vi "ElevatorBegin.vi"(8 "error in (no error)":errorcluster) -> (0 "error out":errorcluster)   [LabVIEW 2023]
doc: "Opens and sets up two SPARK Max Motor Controllers and two limit switches for the Elevator\n\nInputs:\n--Error in--cluster\n\nOutputs:\n--Error out--cluster"
uses:
  <vilib>/Rock Robotics/SystemInterfaces/DIO/FPGA_DIOChannel.ctl
  <vilib>/Rock Robotics/WPI/ThirdParty/REV Robotics/REVLib/Typedef/Spark MAX Limit Switch Polarity.ctl
  <vilib>/Rock Robotics/WPI/ThirdParty/REV Robotics/REVLib/Typedef/Spark MAX Limit Direction.ctl
  <vilib>/Rock Robotics/WPI/ThirdParty/REV Robotics/REVLib/Typedef/Spark MAX Idle Mode.ctl
  <vilib>/Rock Robotics/WPI/ThirdParty/REV Robotics/REVLib/Typedef/Spark MAX Motor Type.ctl
  <vilib>/Rock Robotics/WPI/ThirdParty/REV Robotics/REVLib/Typedef/Spark MAX Sensor Type.ctl
  <vilib>/Rock Robotics/WPI/Switch/WPI_SwitchOpenLimit.vi
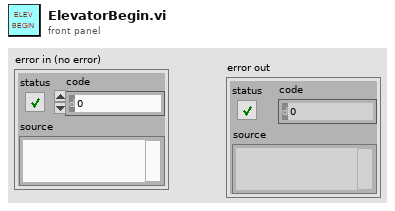
[diagram p1: front panel]
types:
  T1 = typedef "FPGA_DIOChannel.ctl" = enum8{"DIO 0", "DIO 1", "DIO 2", "DIO 3", "DIO 4", "DIO 5", "DIO 6", "DIO 7", "DIO 8", "DIO 9", "DIO MXP 0", "DIO MXP 1", "DIO MXP 2", "DIO MXP 3", "DIO MXP 4", "DIO MXP 5", "DIO MXP 6", "DIO MXP 7", "DIO MXP 8", "DIO MXP 9", "DIO MXP 10", "DIO MXP 11", "DIO MXP 12", "DIO MXP 13", "DIO MXP 14", "DIO MXP 15", "SPI Port CS1", "SPI Port CS2", "SPI Port CS3", "SPI Port MISO", "SPI Port MOSI", "Invalid"}
  T2 = typedef "Spark MAX Limit Switch Polarity.ctl" = enum16{"Normally Open", "Normally Closed"}
  T3 = typedef "Spark MAX Limit Direction.ctl" = enum16{"Forward Limit", "Reverse Limit"}
  T4 = typedef "Spark MAX Idle Mode.ctl" = enum16{"Coast", "Brake"}
  T5 = typedef "Spark MAX Motor Type.ctl" = enum16{"Brushed", "Brushless"}
  T6 = typedef "Spark MAX Sensor Type.ctl" = enum16{"No Sensor", "Hall Sensor", "Encoder", "-Not Available-", "Analog", "Alternate Encoder", "Duty Cycle"}
  T7 = typedef "WPI_MotorControlDeviceRef.ctl" = cluster{"DeviceStatus":errorcluster, "Type":T8, "PWM":cluster{"PWM Channel":T9, "DeadBand":T10}, "CAN":cluster{"Device Number":u8, "SetOutput VI Ref":variant, "GetOutput VI Ref":variant, "Enable VI Ref":variant, "Disable VI Ref":variant, "Data":variant}, "Invert":bool, "DIO PWM":cluster{"PWM \"Enable\" Channel":T9, "DIOChannel":T1, "PWM Rate":dbl}}
  T8 = typedef "WPI_MotorControlType.ctl" = enum16{"PWM", "CAN", "DIO PWM"}
  T9 = typedef "FPGA_DIOPWMChannel.ctl" = enum8{"PWM 0", "PWM 1", "PWM 2", "PWM 3", "PWM 4", "PWM 5", "PWM 6", "PWM 7", "PWM 8", "PWM 9", "PWM MXP 0", "PWM MXP 1", "PWM MXP 2", "PWM MXP 3", "PWM MXP 4", "PWM MXP 5", "PWM MXP 6", "PWM MXP 7", "PWM MXP 8", "PWM MXP 9", "Invalid"}
  T10 = typedef "WPI_PWMDeadband.ctl" = cluster{"Name":string, "maxPositivePwm":i32, "minPositivePwm":i32, "centerPwm":i32, "maxNegativePwm":i32, "minNegativePwm":i32, "angularRange":u16}
  T11 = typedef "WPI_SwitchDevRef.ctl" = cluster{"DevStatus":errorcluster, "DIO Channel":T1, "CntIndex":T12, "Normally Closed":bool}
  T12 = typedef "FPGA_CounterCtrSystemIndex.ctl" = enum8{"Ctr 0", "Ctr 1", "Ctr 2", "Ctr 3", "Ctr 4", "Ctr 5", "Ctr 6", "Ctr 7", "Invalid"}
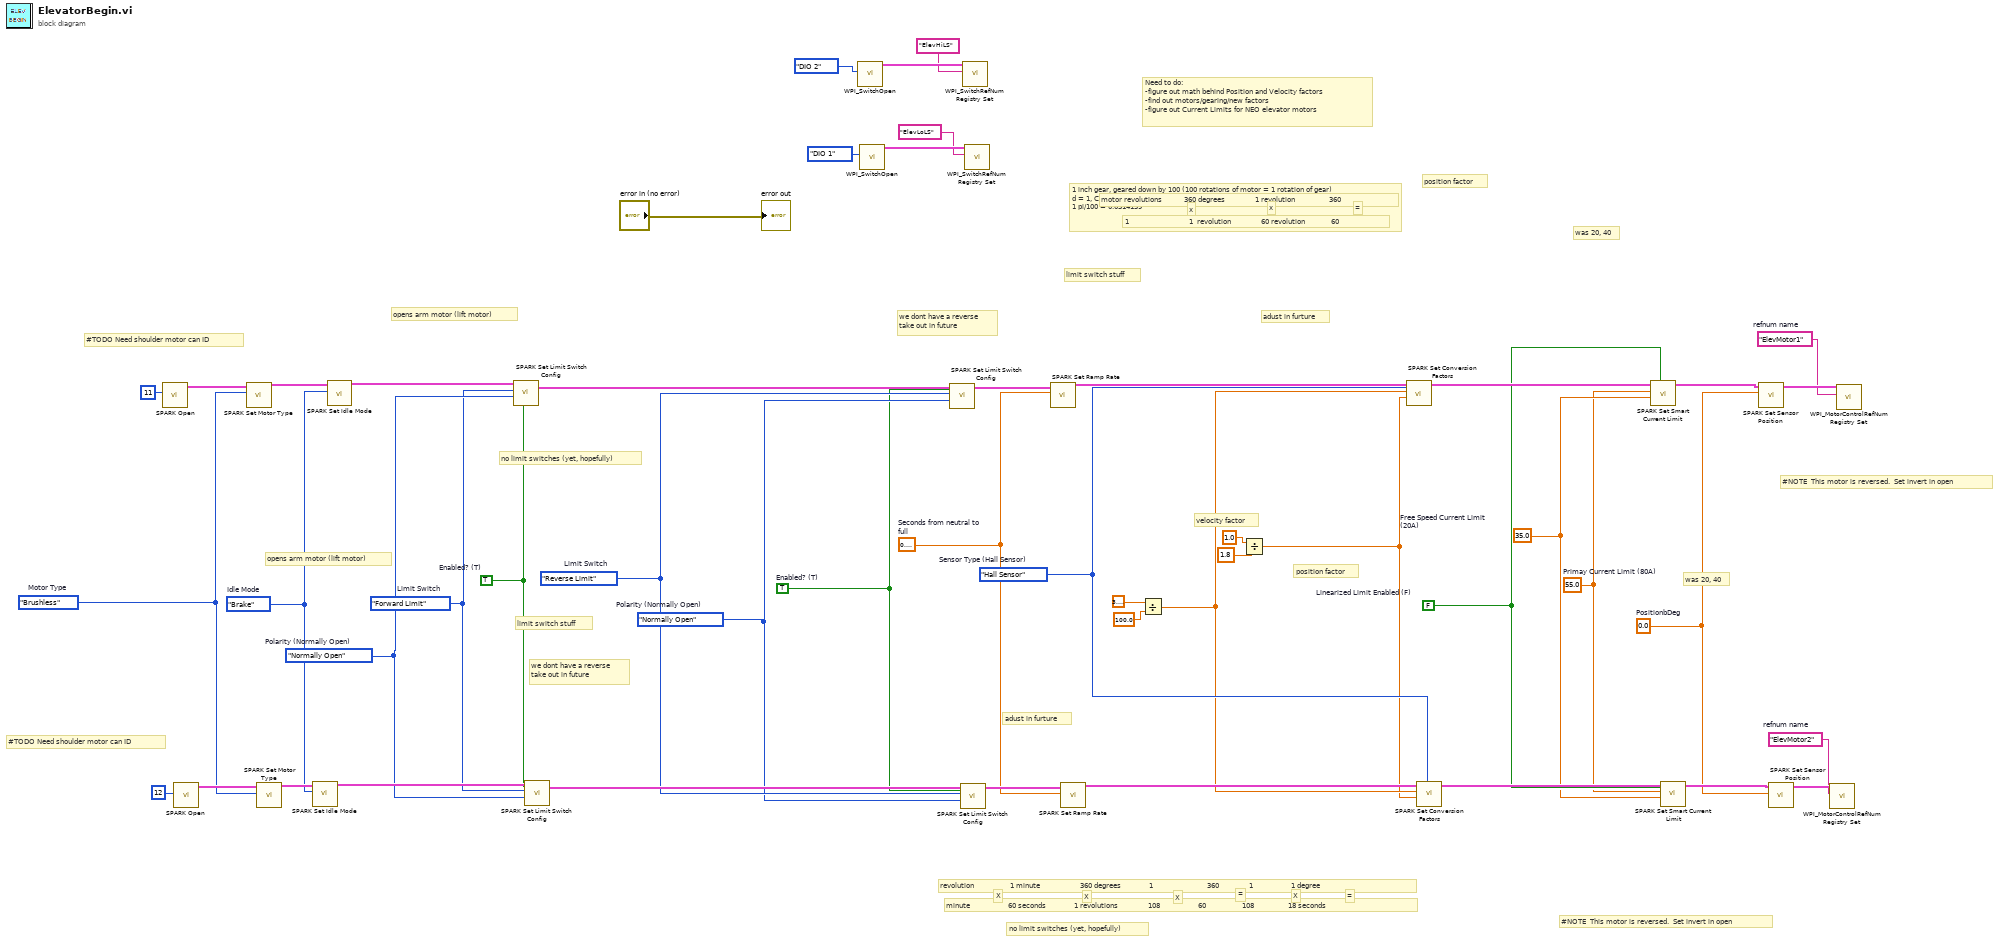
[diagram p0: block diagram]
diagram:
  w4 = FALSE  # Linearized Limit Enabled (F)
  w10 = Spark_MAX_Limit_Switch_Polarity."Normally Open"  # Polarity (Normally Open)
  w11 = Spark_MAX_Limit_Direction."Reverse Limit"  # Limit Switch
  w14 = Spark_MAX_Limit_Switch_Polarity."Normally Open"  # Polarity (Normally Open)
  w13 = Spark_MAX_Limit_Direction."Forward Limit"  # Limit Switch
  w1 = 0.0  # PositionbDeg
  w28 = "ElevMotor2"  # refnum name
  w2 = 55.0  # Primay Current Limit (80A)
  w15 = Spark_MAX_Idle_Mode."Brake"  # Idle Mode
  w16 = Spark_MAX_Motor_Type."Brushless"  # Motor Type
  w7 = Spark_MAX_Sensor_Type."Hall Sensor"  # Sensor Type (Hall Sensor)
  w8 = sgl 0.2  # Seconds from neutral to full
  w9 = TRUE  # Enabled? (T)
  w12 = TRUE  # Enabled? (T)
  w40 = "ElevMotor1"  # refnum name
  w3 = 35.0  # Free Speed Current Limit (20A)
  # "1 inch gear, geared down by 100 (100 rotations of motor = 1 rotation of gear)\nd = 1, C = pi*d = 1pi\n1 pi/100 = 0.0314159"
  # "Need to do: \n-figure out math behind Position and Velocity factors\n-find out motors/gearing/new factors\n-figure out Current Limits for NEO elevator motors"
  # "#NOTE  This motor is reversed.  Set invert in open"
  # "#TODO Need shoulder motor can ID"
  # "no limit switches (yet, hopefully)"
  # "was 20, 40"
  # "we dont have a reverse\ntake out in future"
  # "adust in furture"
  # "position factor"
  # "limit switch stuff"
  # "X"
  # "X"
  # "X"
  # "X"
  # "="
  # "="
  # "minute                   60 seconds              1 revolutions               108                   60                  108                 18 seconds"
  # "revolution                  1 minute                    360 degrees              1                           360               1                   1 degree"
  # "opens arm motor (lift motor)"
  # "#NOTE  This motor is reversed.  Set invert in open"
  # "#TODO Need shoulder motor can ID"
  # "no limit switches (yet, hopefully)"
  # "was 20, 40"
  # "we dont have a reverse\ntake out in future"
  # "adust in furture"
  # "velocity factor"
  # "position factor"
  # "limit switch stuff"
  # "1                              1  revolution               60 revolution             60"
  # "="
  # "x"
  # "x"
  # "motor revolutions           360 degrees               1 revolution                 360"
  # "opens arm motor (lift motor)"
  n1 = call <vilib>:"SPARK Open.vi"("Device Number"=u8 11) -> ("MotorControlDeviceRef"=w44:T7)  [unwired: 9 in, 1 out]
  n2 = call <vilib>:"SPARK Open.vi"("Device Number"=u8 12) -> ("MotorControlDeviceRef"=w32:T7)  [unwired: 9 in, 1 out]
  n3 = call <vilib>:"SPARK Set Motor Type.vi"("Motor Type"=w16, "MotorControlDevRef"=w44) -> ("MotorControlDeviceRef"=w43:T7)  [unwired: 8 in, 1 out]
  n4 = call <vilib>:"SPARK Set Motor Type.vi"("Motor Type"=w16, "MotorControlDevRef"=w32) -> ("MotorControlDeviceRef"=w31:T7)  [unwired: 8 in, 1 out]
  n5 = call <vilib>:"SPARK Set Idle Mode.vi"("Idle Mode"=w15, "MotorControlDeviceRef in"=w31) -> ("MotorControlDeviceRef out"=w27:T7)  [unwired: 8 in, 1 out]
  n6 = call <vilib>:"SPARK Set Idle Mode.vi"("Idle Mode"=w15, "MotorControlDeviceRef in"=w43) -> ("MotorControlDeviceRef out"=w39:T7)  [unwired: 8 in, 1 out]
  n7 = call <vilib>:"SPARK Set Limit Switch Config.vi"("Enabled? (T)"=w12, "Polarity (Normally Open)"=w14, "Limit Switch"=w13, "MotorControlDeviceRef in"=w39) -> ("MotorControlDeviceRef out"=w38:T7)  [unwired: 6 in, 1 out]
  n8 = call <vilib>:"SPARK Set Limit Switch Config.vi"("Enabled? (T)"=w12, "Polarity (Normally Open)"=w14, "Limit Switch"=w13, "MotorControlDeviceRef in"=w27) -> ("MotorControlDeviceRef out"=w26:T7)  [unwired: 6 in, 1 out]
  n9 = call-poly <vilib>:"WPI_SwitchOpen.vi"("DIO Channel"=FPGA_DIOChannel."DIO 2") -> ("SwitchDevRef"=w48:T11)  [unwired: 9 in, 1 out]
  n10 = call-poly <vilib>:"WPI_SwitchOpen.vi"("DIO Channel"=FPGA_DIOChannel."DIO 1") -> ("SwitchDevRef"=w46:T11)  [unwired: 9 in, 1 out]
  n11 = call <vilib>:"SPARK Set Limit Switch Config.vi"("Enabled? (T)"=w9, "Polarity (Normally Open)"=w10, "Limit Switch"=w11, "MotorControlDeviceRef in"=w38) -> ("MotorControlDeviceRef out"=w37:T7)  [unwired: 6 in, 1 out]
  n12 = call <vilib>:"SPARK Set Limit Switch Config.vi"("Enabled? (T)"=w9, "Polarity (Normally Open)"=w10, "Limit Switch"=w11, "MotorControlDeviceRef in"=w26) -> ("MotorControlDeviceRef out"=w25:T7)  [unwired: 6 in, 1 out]
  n13 = call <vilib>:"WPI_SwitchRefNum Registry Set.vi"("refnum name"="ElevHiLS", "SwitchDevRef"=w48) -> ()  [unwired: 8 in, 2 out]
  n14 = call <vilib>:"WPI_SwitchRefNum Registry Set.vi"("refnum name"="ElevLoLS", "SwitchDevRef"=w46) -> ()  [unwired: 8 in, 2 out]
  n15 = call <vilib>:"SPARK Set Ramp Rate.vi"("Seconds from neutral to full (0)"=w8, "MotorControlDeviceRef in"=w37) -> ("MotorControlDeviceRef"=w36:T7)  [unwired: 8 in, 1 out]
  n16 = call <vilib>:"SPARK Set Ramp Rate.vi"("Seconds from neutral to full (0)"=w8, "MotorControlDeviceRef in"=w25) -> ("MotorControlDeviceRef"=w24:T7)  [unwired: 8 in, 1 out]
  n17 = Divide(x=3.141592653589793, y=100.0) -> (x/y=w6:dbl)
  n18 = Divide(x=1.0 ("Velocity Factor (1)"), y=1.8) -> (x/y=w5:dbl)
  n19 = call <vilib>:"SPARK Set Conversion Factors.vi"("Sensor Type (Hall Sensor)"=w7, "Velocity Factor (1)"=w5, "Position Factor (1)"=w6, "MotorControlDeviceRef in"=w36) -> ("MotorControlDeviceRef out"=w35:T7)  [unwired: 6 in, 1 out]
  n20 = call <vilib>:"SPARK Set Conversion Factors.vi"("Sensor Type (Hall Sensor)"=w7, "Velocity Factor (1)"=w5, "Position Factor (1)"=w6, "MotorControlDeviceRef in"=w24) -> ("MotorControlDeviceRef out"=w23:T7)  [unwired: 6 in, 1 out]
  n21 = call <vilib>:"SPARK Set Smart Current Limit.vi"("Linearized Limit Enabled (F)"=w4, "Free Speed Current Limit (20A)"=w3, "Primay Current Limit (80A)"=w2, "MotorControlDeviceRef in"=w35) -> ("MotorControlDeviceRef out"=w42:T7)  [unwired: 6 in, 1 out]
  n22 = call <vilib>:"SPARK Set Smart Current Limit.vi"("Linearized Limit Enabled (F)"=w4, "Free Speed Current Limit (20A)"=w3, "Primay Current Limit (80A)"=w2, "MotorControlDeviceRef in"=w23) -> ("MotorControlDeviceRef out"=w30:T7)  [unwired: 6 in, 1 out]
  n23 = call <vilib>:"SPARK Set Sensor Position.vi"("Position"=w1, "MotorControlDeviceRef"=w42) -> ("MotorControlDeviceRef"=w41:T7)  [unwired: 8 in, 1 out]
  n24 = call <vilib>:"SPARK Set Sensor Position.vi"("Position"=w1, "MotorControlDeviceRef"=w30) -> ("MotorControlDeviceRef"=w29:T7)  [unwired: 8 in, 1 out]
  n25 = call <vilib>:"WPI_MotorControlRefNum Registry Set.vi"("refnum name"=w28, "MotorControlDevRef"=w29) -> ()  [unwired: 8 in, 2 out]
  n26 = call <vilib>:"WPI_MotorControlRefNum Registry Set.vi"("refnum name"=w40, "MotorControlDevRef"=w41) -> ()  [unwired: 8 in, 2 out]
  "error out" <- "error in (no error)"
